vi "ALTS-2015 LV2GBL Queue.vi"(6 "Enum":enum16{"Init", "Enqueue", "Dequeue", "Destroy"}(ring), 8 "error in (no error)":errorcluster, 10 "Enqueue Element":cluster{"Test Status":string, "Station Name":T1}, 11 "Queue name":string) -> (0 "error out":errorcluster, 3 "Dequeued Element":cluster{"Test Status":string, "Station Name":T1})   [LabVIEW 2013]
uses:
  Controls/ALTS-2015 Station Cluster.ctl
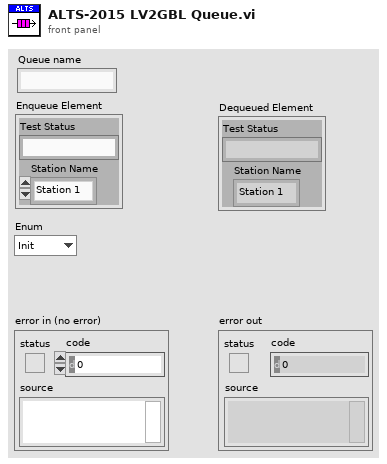
[diagram p1: front panel]
types:
  T1 = typedef "ALTS-2015 Station Cluster.ctl" = enum16{"Station 1", "Station 2", "Station 3", "Station 4"}
  T2 = cluster{"Test Status":string, "deleted portion":T1}
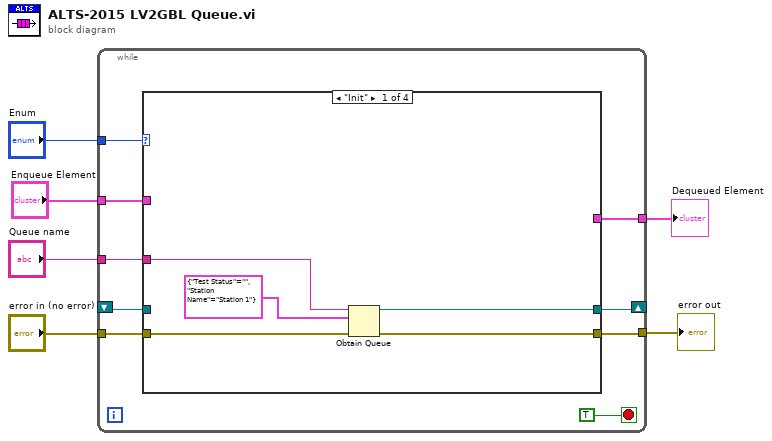
[diagram p0: block diagram]
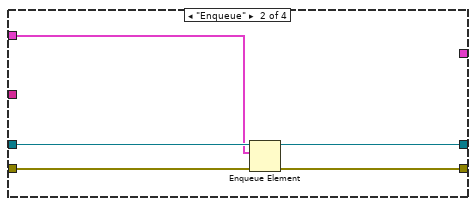
[diagram p2: hidden frame]
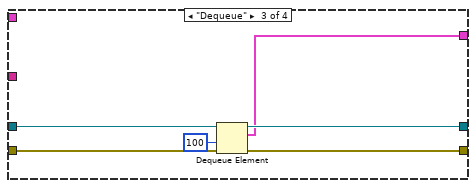
[diagram p3: hidden frame]
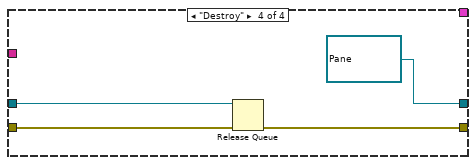
[diagram p4: hidden frame]
diagram:
  n1 = while {
    tunnel: "Enum" -> [w15]
    tunnel: "error in (no error)" -> [w13]
    tunnel: [w12] -> w4
    tunnel: "Queue name" -> [w11]
    shift-right: [w10] -> _
    shift-left: _ -> [w8]
    tunnel: "Enqueue Element" -> [w9]
    tunnel: [w7] -> w1
    stop <- TRUE stop-if-true
    n2 = case shown="\"Init\"" w15 {
      tunnel: w13 -> [w20 w25 w31 w35]
      tunnel: [w19 w22 w28 w33] -> w12
      tunnel: w11 -> [w18 _ _ _]
      tunnel: [w17 w23 w27 refnum<queue> refnum ("queue out")] -> w10
      tunnel: w9 -> [_ w21 _ _]
      tunnel: w8 -> [_ w24 w30 w34]
      tunnel: [_ _ w26 _] -> w7
      frame "Init" {
        n3 = Obtain Queue(name (unnamed)=w18, element data type=cluster{"Test Status":string, "Station Name":T1} {"Test Status"="", "Station Name"=enum."Station 1"} ("Enqueue Element"), error in (no error)=w20) -> (queue out=w17:refnum<queue>, error out=w19:errorcluster)  [unwired: 2 in, 1 out]
      }
      frame "Enqueue" {
        n4 = Enqueue Element(queue=w24, element=w21, error in (no error)=w25) -> (queue out=w23:refnum<queue>, error out=w22:errorcluster)  [unwired: 1 in, 1 out]
      }
      frame "Dequeue" {
        n5 = Dequeue Element(queue=w30, timeout in ms (-1)=100, error in (no error)=w31) -> (queue out=w27:refnum<queue>, element=w26:T2, error out=w28:errorcluster)  [unwired: 1 out]
      }
      frame "Destroy" {
        n6 = Release Queue(queue=w34, error in (no error)=w35) -> (error out=w33:errorcluster)  [unwired: 1 in, 2 out]
      }
    }
  }
  "error out" <- w4
  "Dequeued Element" <- w1
